vi "Operation to Machine Job Tuple.vi"(9 "Number of Machines":i32, 11 "Operation Number":i32) -> (1 "Job No":i32, 3 "Machine No":i32)   [LabVIEW 2013, in "GanntChart.lvclass"]
uses:
  GanntChart.lvclass
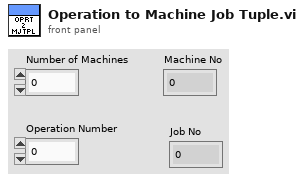
[diagram p1: front panel]
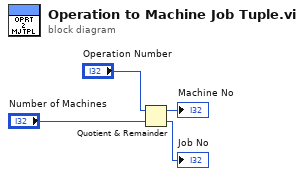
[diagram p0: block diagram]
diagram:
  n1 = Quotient & Remainder(x="Operation Number", y="Number of Machines") -> (x-y*floor(x/y)=→"Machine No":i32, floor(x/y)=→"Job No":i32)
